vi "SS Calculate.vi"(6 "index":i32, 8 "error in (no error)":errorcluster, 10 "SS measurement":T1={"Signal frequencies (Hz)"=[1000.0], "Signal amplitudes (V)"=[0.707], "Sampling frequencies (Hz)"=[10000000.0], "Record lengths (multiples of periods)"=[10000.0], "Calculate results"=FALSE, "Algorithm"="TWM-PJVSSubS", "TWM data directories"=[], "TWM data directories relative"=[], "Settle down after AC source change (s)"=1.0, "PJVS frequencies (Hz)"=[1000.0], "PJVS reference voltages array of vector cluster"=[{"PJVS reference voltages vector"=[]}], "Requested PJVS steps"=[20], "Measure CE"=FALSE, "Measure CE before"=FALSE, "Measure CE after"=FALSE, "Single point CE measurement"=FALSE, "original CE template path"=path "", "new CE template path before SS"=path "", "new CE template path before SS relative"=path "", "new CE template path after SS"=path "", "new CE template path after SS relative"=path "", "original CE fit path"=path "", "new CE fit path before SS"=path "", "new CE fit path before SS relative"=path "", "new CE fit path after SS"=path "", "new CE fit path after SS relative"=path "", "Measure digitizer gain"=FALSE, "Measure digitizer gain before"=FALSE, "Measure digitizer gain after"=FALSE, "Digitizer gain"=0.0, "Data folder"=path "", "FR fit path"=path "", "new FR fit path relative"=path "", "Rs"=0, "Re"=0, "SS measurement info files"=[]} {"PJVS reference voltages array of vector cluster"."PJVS reference voltages vector" format="%#_3p"; "PJVS frequencies (Hz)" format="%#_3p"; "Record lengths (multiples of periods)" format="%#_3p"; "Sampling frequencies (Hz)" format="%#_3p"; "Signal amplitudes (V)" format="%#_3p"; "Signal frequencies (Hz)" format="%#_3p"}, 11 "Common properties":T2={"Measurement status ref"=refnum, "TWM Status ref"=refnum, "Abort ref"=refnum, "Skip waiting ref"=refnum, "GNU Octave path"=path "C:/Program Files/GNU Octave/Octave-6.2.0/mingw64/bin", "TWM+QWTB path"=path "C:/Users/labina/Desktop/TWM-1.8.7.0-full/octprog", "lvlib path"=path "D:/martin/WAC/WACsw - github/control_software/Filter function meter/external libraries/GOLPI 0.7.3.1 source distribution LV 20.0 32 bit/lv_proc.dll", "TWM pipe"="\\\\.\\pipe\\TWM:server", "PJVS status ref"=refnum, "WAC path"=path ""}) -> (0 "error out":errorcluster)   [LabVIEW 2020]
doc: "Change octave path, add paths to WAC data processing."
uses:
  Utilities/Type definitions/Common properties.ctl
  SS Measurement/Type definitions/SS measurement.ctl
  Utilities/Calculation related/Globals for GOLPI.vi
  external libraries/GOLPI 0.7.3.1 source distribution LV 20.0 32 bit/GOLPI library.lvlib
panel:
  out "command\n(for debug)":string="addpath('info'); addpath('qwtb'); qwtb_exec_algorithm('%s', 0, 1); disp('FINISHEDCR')"
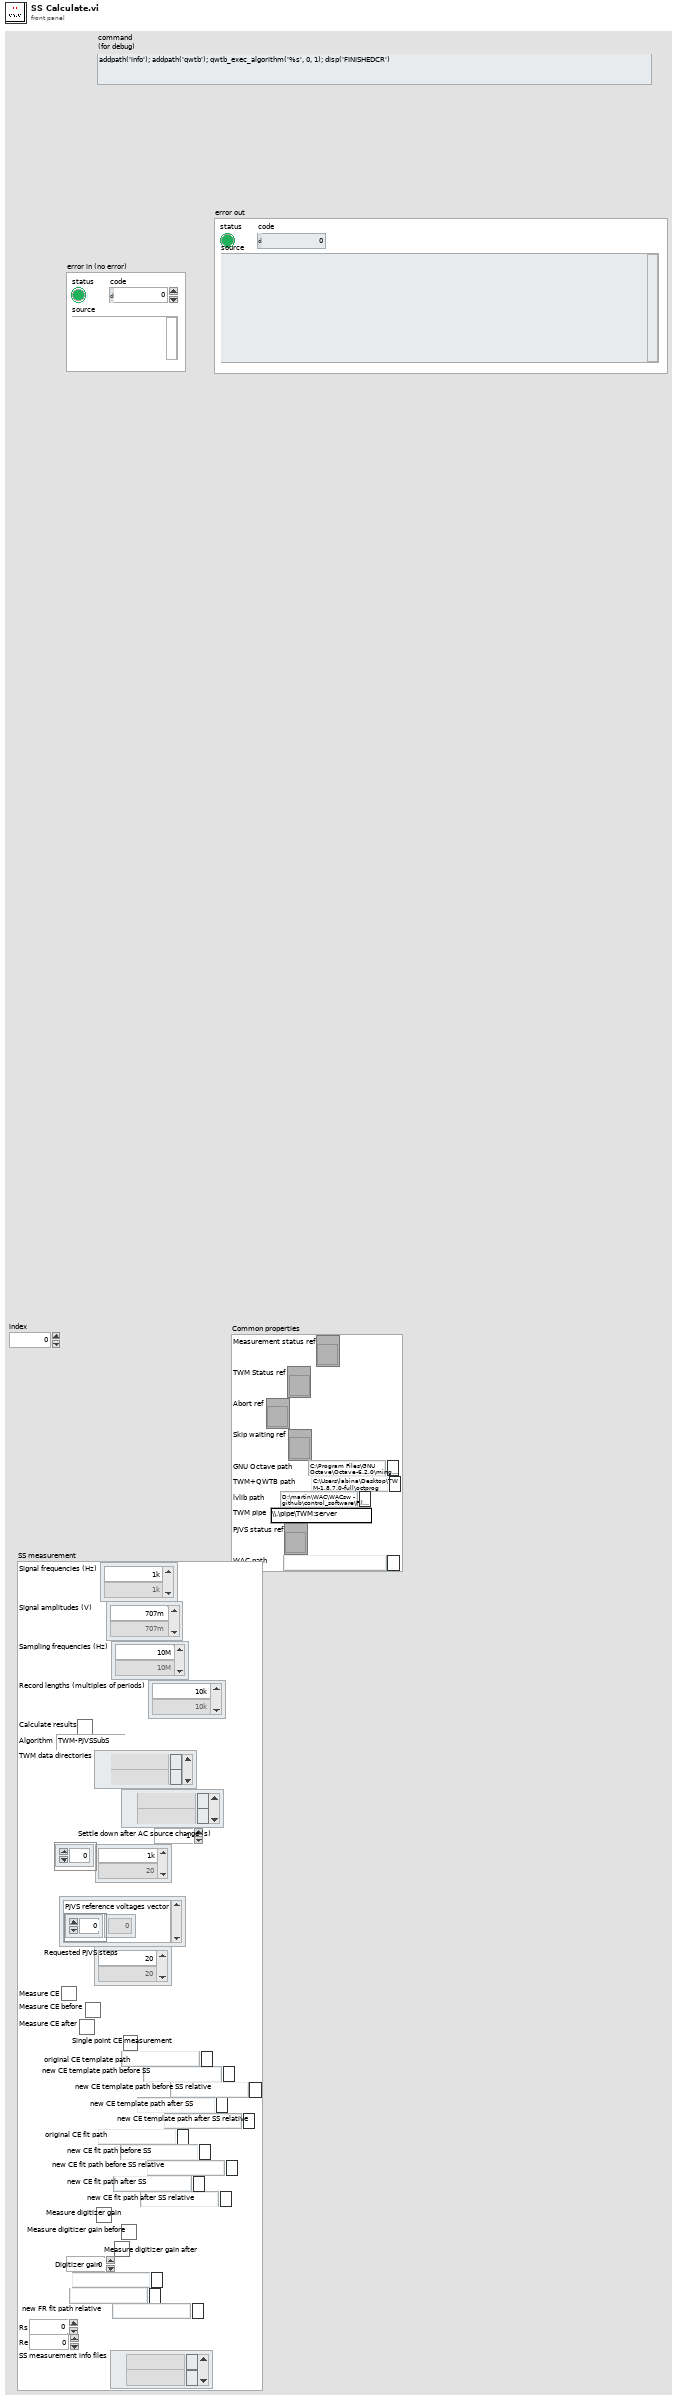
[diagram p1: front panel]
types:
  T1 = typedef "SS measurement.ctl" = cluster{"Signal frequencies (Hz)":dbl[], "Signal amplitudes (V)":dbl[], "Sampling frequencies (Hz)":dbl[], "Record lengths (multiples of periods)":dbl[], "Calculate results":bool, "Algorithm":string, "TWM data directories":path[], "TWM data directories relative":path[], "Settle down after AC source change (s)":dbl, "PJVS frequencies (Hz)":dbl[], "PJVS reference voltages array of vector cluster":cluster{"PJVS reference voltages vector":dbl[]}[], "Requested PJVS steps":u32[], "Measure CE":bool, "Measure CE before":bool, "Measure CE after":bool, "Single point CE measurement":bool, "original CE template path":path, "new CE template path before SS":path, "new CE template path before SS relative":path, "new CE template path after SS":path, "new CE template path after SS relative":path, "original CE fit path":path, "new CE fit path before SS":path, "new CE fit path before SS relative":path, "new CE fit path after SS":path, "new CE fit path after SS relative":path, "Measure digitizer gain":bool, "Measure digitizer gain before":bool, "Measure digitizer gain after":bool, "Digitizer gain":dbl, "Data folder":path, "FR fit path":path, "new FR fit path relative":path, "Rs":i32, "Re":i32, "SS measurement info files":path[]}
  T2 = typedef "Common properties.ctl" = cluster{"Measurement status ref":refnum<vi>, "TWM Status ref":refnum<vi>, "Abort ref":refnum<vi>, "Skip waiting ref":refnum<vi>, "GNU Octave path":path, "TWM+QWTB path":path, "lvlib path":path, "TWM pipe":string, "PJVS status ref":refnum<vi>, "WAC path":path}
  T3 = typedef "GOLPI library.lvlib/GOLPI reference Type Def.ctl" = cluster{"pipe handle":T4, "fast read timeout [ms]":u32, "fast read settle time [ms]":u32, "fast read to multiple [ms]":u32, "max elements per input line":u32, "slow read timeout [ms]":u32, "stdin double format specifier":string, "max elements per stdout output column":u32, "console mode bitstream":bool, "bitstream first read timeout [ms]":u32, "bitstream read timeout [ms]":u32, "struct transfer possible":bool, "matlab mode":bool}
  T4 = typedef "LV Process library.lvlib/Pipe Handle.ctl" = cluster{"lv_proc.dll file path":path, "process instance handle":u32[], "debug mode":bool, "debug data":cluster{"time":timestamp, "stdin":bool, "data":string}[]}
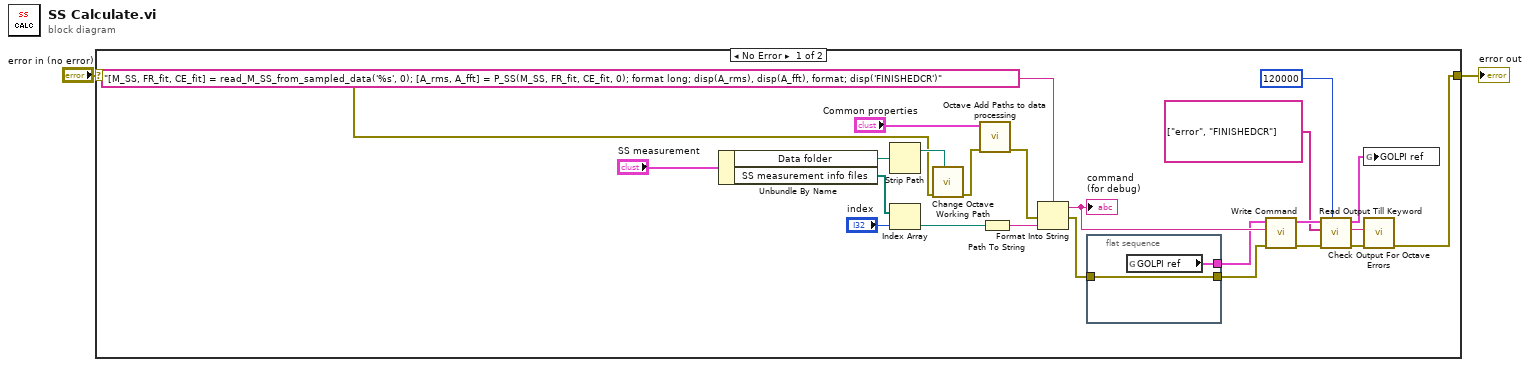
[diagram p0: block diagram]
diagram:
  n1 = case shown="No Error" "error in (no error)" {
    selector: "error in (no error)" -> [w18 w29]
    tunnel: [w8 w29] -> w2
    frame No Error {
      n2 = Unbundle By Name("SS measurement") -> ("Data folder"=w17:path, "SS measurement info files"=w5:path[])
      n3 = Strip Path(path=w17) -> (stripped path=w19:path)  [unwired: 1 out]
      n4 = Index Array(array=w5, index="index") -> (element=w4:path)
      n5 = call "Change Octave Working Path.vi"("Measurement path in"=w19, "error in (no error)"=w18) -> ("error out"=w12:errorcluster)  [unwired: 9 in]
      n6 = call "Octave Add Paths to data processing.vi"("error in (no error)"=w12, "Common properties"="Common properties") -> ("error out"=w11:errorcluster)  [unwired: 9 in]
      n7 = Path To String(path=w4) -> (string=w25:string)
      n8 = Format Into String(format string="[M_SS, FR_fit, CE_fit] = read_M_SS_from_sampled_data('%s', 0); [A_rms, A_fft] = P_SS(M_SS, FR_fit, CE_fit, 0); format long; disp(A_rms), disp(A_fft), format; disp('FINISHEDCR')", error in=w11, w25) -> (resulting string=w20:string, error out=w16:errorcluster)  [unwired: 1 in]
      "command\n(for debug)" <- w20
      n9 = flat-sequence {
        tunnel: [w28] -> w15
        tunnel: w16 -> [w28]
        tunnel: [w27] -> w14
        frame #0 {
          n10 = global read "Globals for GOLPI.vi" "GOLPI ref"() -> (w27:T3)
        }
      }
      n11 = call "Write Command.vi"("error in"=w15, "command"=w20, "GOLPI ref. in"=w14) -> ("error out"=w24:errorcluster, "GOLPI ref. out"=w23:T3)  [unwired: 7 in]
      n12 = call "Read Output Till Keyword.vi"("timeout [ms]"=u32 120000, "error in"=w24, "keywords"=string[] ["error", "FINISHEDCR"], "GOLPI ref. in"=w23) -> ("error out"=w9:errorcluster, "read buffer"=w7:string, "GOLPI ref. out"=w13:T3)  [unwired: 4 in, 1 out]
      n13 = global write "Globals for GOLPI.vi" "GOLPI ref"(w13) -> ()
      n14 = call "Check Output For Octave Errors.vi"("error in"=w9, "read buffer"=w7) -> ("error out"=w8:errorcluster)  [unwired: 9 in]
    }
    frame Error {
    }
  }
  "error out" <- w2
